vi "test - LabVIEW-Config Read Array.vi"(8 "error in (no error)":errorcluster, 11 "TestCase in":refnum<class "labview-config-library.lvclass">) -> (0 "error out":errorcluster, 3 "TestCase out":refnum<class "labview-config-library.lvclass">)   [LabVIEW 2017, in "labview-config-library.lvclass"]
uses:
  labview-config-library.lvclass
  <vilib>/addons/_JKI Toolkits/VI Tester/TestCase.llb/TestCase.lvclass
  C:/Program Files (x86)/National Instruments/LabVIEW 2017/vi.lib/addons/_JKI Toolkits/VI Tester/TestCase.llb/TestCase.lvclass
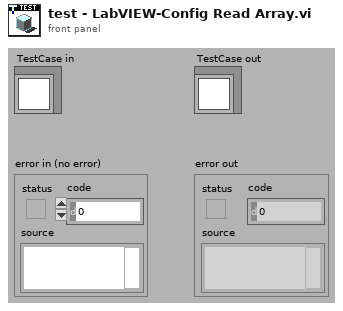
[diagram p1: front panel]
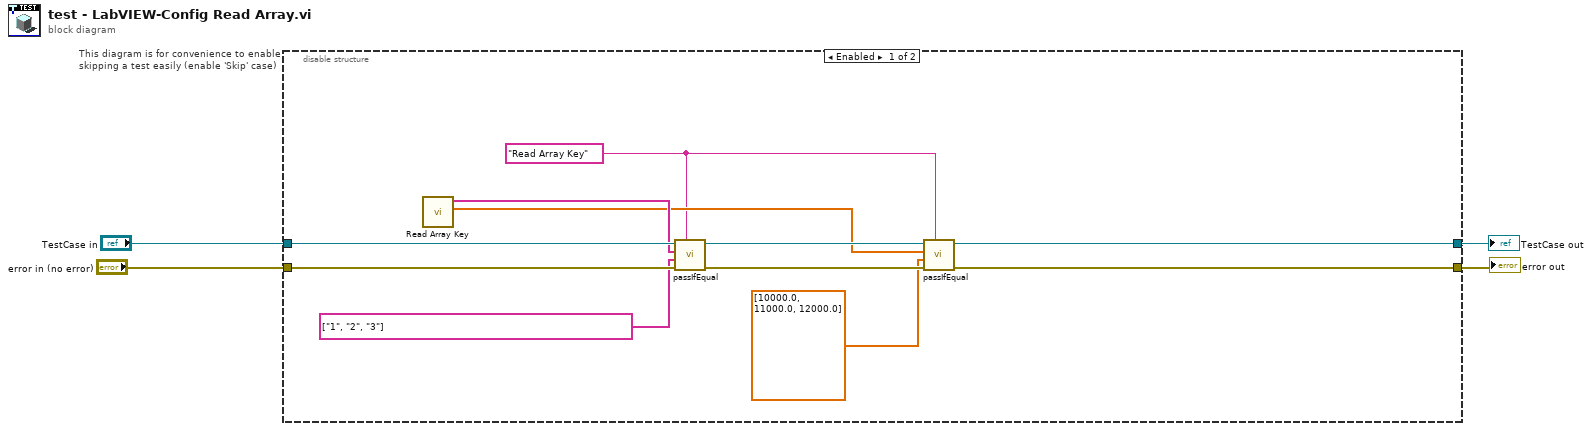
[diagram p0: block diagram]
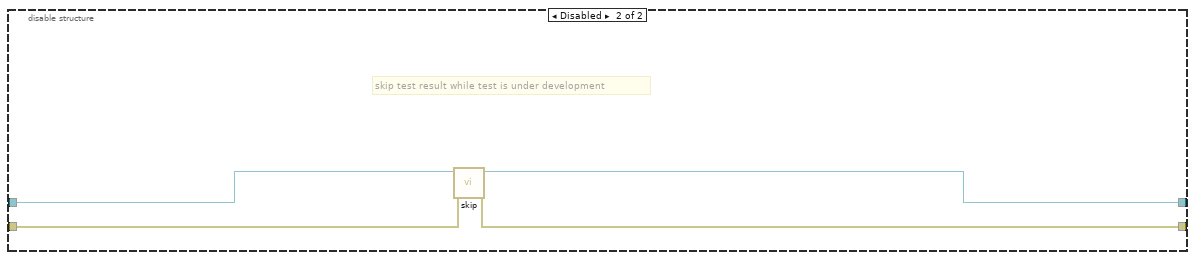
[diagram p2: hidden frame]
diagram:
  n1 = disable-structure "This diagram is for convenience to enable skipping a test easily (enable 'Skip' case)" shown="Enabled" {
    disable-tunnel: "TestCase in" -> [w15 w19]
    disable-tunnel: [w11 w17] -> w1
    disable-tunnel: [w10 w18] -> w3
    disable-tunnel: "error in (no error)" -> [w14 w16]
    frame Enabled {
      w7 = "Read Array Key" ("custom report message (\"\")")
      n2 = call "Read Array Key.vi"() -> ("def"=w8:dbl[], "abc"=w9:string[])  [unwired: 10 in]
      n3 = call-dynamic "passIfEqual.vi"("custom report message (\"\")"=w7, "error in (no error)"=w14, "y"=string[] ["1", "2", "3"] ("abc"), "x"=w9, "TestCase in"=w15) -> ("error out"=w13:errorcluster, "TestCase out"=w12:refnum<class "labview-config-library.lvclass">)  [unwired: 5 in]
      n4 = call-dynamic "passIfEqual.vi"("custom report message (\"\")"=w7, "error in (no error)"=w13, "y"=dbl[] [10000.0, 11000.0, 12000.0] ("def"), "x"=w8, "TestCase in"=w12) -> ("error out"=w10:errorcluster, "TestCase out"=w11:refnum<class "labview-config-library.lvclass">)  [unwired: 5 in]
    }
    frame Disabled {
      # "skip test result while test is under development"
      n5 = call <vilib>:"skip.vi"("error in (no error)"=w16, "TestCase in"=w19) -> ("error out"=w18:errorcluster, "TestCase out"=w17:refnum<class "labview-config-library.lvclass">)  [unwired: 8 in]
    }
  }
  "error out" <- w3
  "TestCase out" <- w1
